vi "controlActorSelection.vi"(7 "set":bool, 8 "error in":errorcluster, 9 "Positioner in":string, 10 "axis":u8(ring) items=["1", "2", "3"]) -> (0 "error out":errorcluster, 1 "Positioner out":string, 2 "axis out":u8, 4 "allPositioners":string[](array[string]))   [LabVIEW 2016]
panel:
  in  "connection ID":refnum<k5>
  out "connection ID out":refnum<k5>
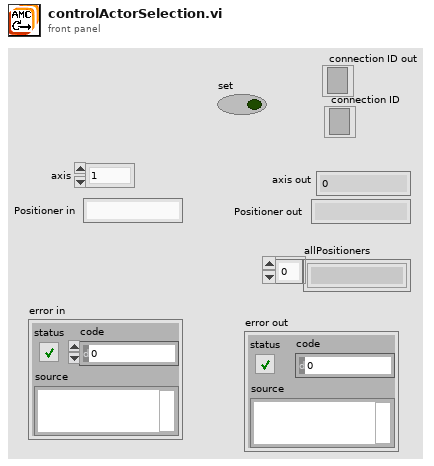
[diagram p1: front panel]
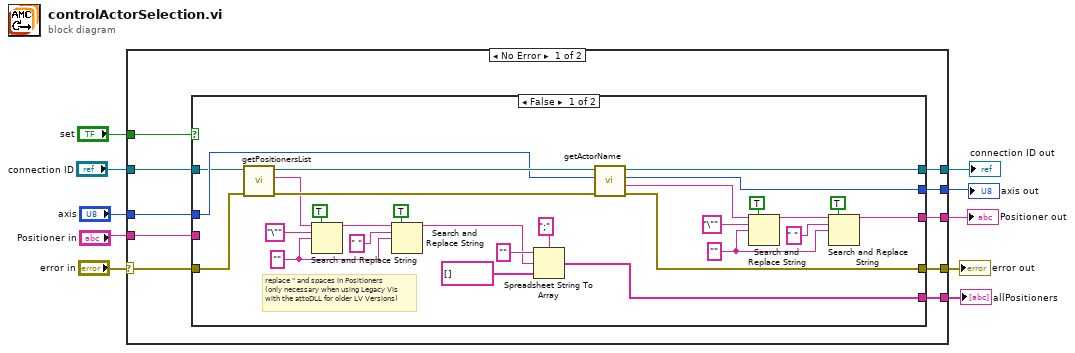
[diagram p0: block diagram]
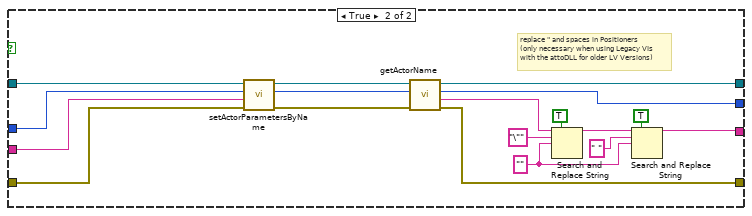
[diagram p2: hidden frame]
diagram:
  n1 = case shown="No Error" "error in" {
    selector: "error in" -> [w19 w68]
    tunnel: "axis" -> [w17 w69]
    tunnel: [w18 w68] -> w10
    tunnel: [w16 w69] -> w9
    tunnel: "Positioner in" -> [w15 w67]
    tunnel: [w20 w70] -> w2
    tunnel: "set" -> [w14 _]
    tunnel: [w13 w67] -> w5
    tunnel: [w12 _] -> w4
    tunnel: "connection ID" -> [w11 _]
    frame No Error {
      n2 = case shown="False" w14 {
        tunnel: [w48 w62] -> w20
        tunnel: w19 -> [w40 w66]
        tunnel: [w46 w60] -> w18
        tunnel: w17 -> [w41 w65]
        tunnel: [w47 w58] -> w16
        tunnel: w15 -> [_ w64]
        tunnel: [w22 w50] -> w13
        tunnel: [w38 _] -> w12
        tunnel: w11 -> [w21 w49]
        frame False {
          w26 = "" ("replace string (\"\")")
          w32 = "" ("replace string (\"\")")
          # "replace \" and spaces in Positioners\n(only necessary when using Legacy VIs\nwith the attoDLL for older LV Versions)"
          n3 = call "getPositionersList.vi"("error in"=w40, "connection ID"=w21) -> ("error out"=w39:errorcluster, "PositionersList"=w37:string, "connection ID"=w42:refnum<k5>)  [unwired: 7 in]
          n4 = Search and Replace String(replace all?=TRUE ("replace all? (F)"), input string=w37, search string="\"", replace string=w32) -> (result string=w36:string)  [unwired: 4 in, 3 out]
          n5 = Search and Replace String(replace all?=TRUE ("replace all? (F)"), input string=w36, search string=" ", replace string=w32) -> (result string=w35:string)  [unwired: 4 in, 3 out]
          n6 = Spreadsheet String To Array(delimiter (Tab)=";", format string="", spreadsheet string=w35, array type (2D Dbl)=string[] []) -> (array=w38:string[])
          n7 = call "getActorName.vi"("error in"=w39, "axis"=w41, "connection ID"=w42) -> ("error out"=w46:errorcluster, "actor_name"=w23:string, "axis_out"=w47:i32, "connection ID"=w48:refnum<k5>)  [unwired: 5 in]
          n8 = Search and Replace String(replace all?=TRUE ("replace all? (F)"), input string=w23, search string="\"", replace string=w26) -> (result string=w29:string)  [unwired: 4 in, 3 out]
          n9 = Search and Replace String(replace all?=TRUE ("replace all? (F)"), input string=w29, search string=" ", replace string=w26) -> (result string=w22:string)  [unwired: 4 in, 3 out]
        }
        frame True {
          w54 = "" ("replace string (\"\")")
          # "replace \" and spaces in Positioners\n(only necessary when using Legacy VIs\nwith the attoDLL for older LV Versions)"
          n10 = call "setActorParametersByName.vi"("error in"=w66, "actorname"=w64, "axis"=w65, "connection ID"=w49) -> ("error out"=w61:errorcluster, "axis_out"=w59:i32, "connection ID"=w63:refnum<k5>)  [unwired: 5 in]
          n11 = call "getActorName.vi"("error in"=w61, "axis"=w59, "connection ID"=w63) -> ("error out"=w60:errorcluster, "actor_name"=w51:string, "axis_out"=w58:i32, "connection ID"=w62:refnum<k5>)  [unwired: 5 in]
          n12 = Search and Replace String(replace all?=TRUE ("replace all? (F)"), input string=w51, search string="\"", replace string=w54) -> (result string=w57:string)  [unwired: 4 in, 3 out]
          n13 = Search and Replace String(replace all?=TRUE ("replace all? (F)"), input string=w57, search string=" ", replace string=w54) -> (result string=w50:string)  [unwired: 4 in, 3 out]
        }
      }
    }
    frame Error {
    }
  }
  "error out" <- w10
  "axis out" <- w9
  "Positioner out" <- w5
  "allPositioners" <- w4
  "connection ID out" <- w2
